vi "Decode.vi"(2 "Measurements":dbl[](array[numeric]), 8 "error in (no error)":errorcluster, 10 "Input String":string, 11 "IMU in":refnum<class "IMU.lvclass">) -> (0 "error out":errorcluster, 3 "IMU out":refnum<class "IMU.lvclass">)   [LabVIEW 2021, in "IMU.lvclass"]
uses:
  IMU.lvclass
  IMU.lvclass/IMU.ctl
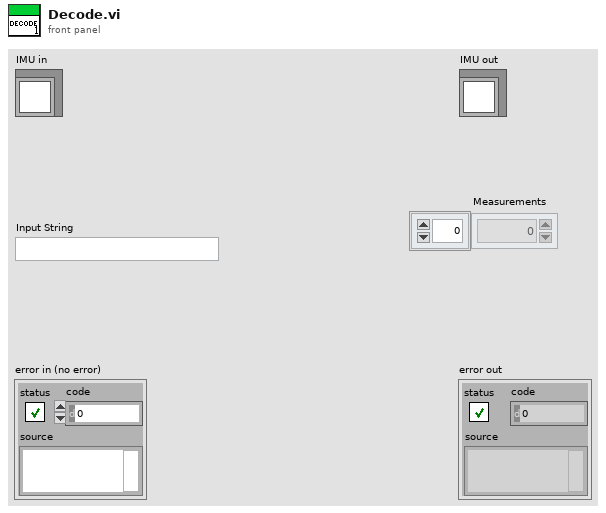
[diagram p1: front panel]
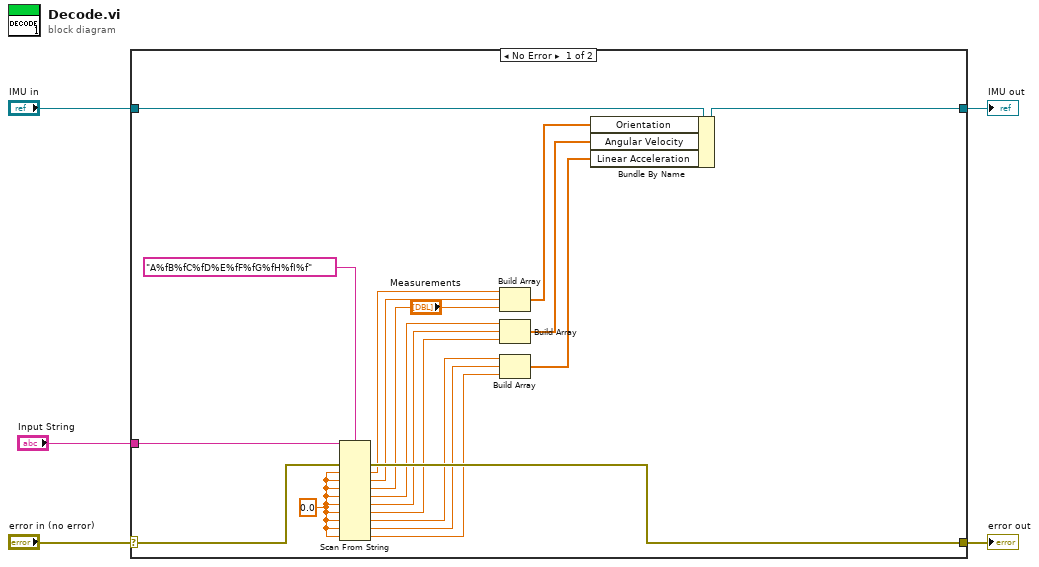
[diagram p0: block diagram]
diagram:
  n1 = case shown="No Error" "error in (no error)" {
    selector: "error in (no error)" -> [w22 w26]
    tunnel: [w21 w26] -> w4
    tunnel: [w19 w25] -> w2
    tunnel: "IMU in" -> [w20 w25]
    tunnel: "Input String" -> [w24 _]
    frame No Error {
      w18 = 0.0
      n2 = Scan From String(format string="A%fB%fC%fD%E%fF%fG%fH%fI%f" ("regular expression"), input string=w24, error in=w22, default 1=w18, default 2=w18, default 3=w18, default 4=w18, default 5=w18, default 6=w18, default 7=w18, default 8=w18, default 9=w18) -> (error out=w21:errorcluster, output 1=w17:dbl, output 2=w16:dbl, output 3=w15:dbl, output 4=w14:dbl, output 5=w13:dbl, output 6=w12:dbl, output 7=w11:dbl, output 8=w10:dbl, output 9=w9:dbl)  [unwired: 1 in, 2 out]
      n3 = Build Array(w17, w16, w15) -> (w8:dbl[])
      n4 = Build Array(w14, w13, w12) -> (w7:dbl[])
      n5 = Build Array(w11, w10, w9) -> (w6:dbl[])
      n6 = Bundle By Name(cluster=w20, "Orientation"=w8, "Angular Velocity"=w7, "Linear Acceleration"=w6) -> (w19:refnum<class "IMU.lvclass">)
    }
    frame Error {
    }
  }
  "error out" <- w4
  "IMU out" <- w2
